vi "Reset.vi"(8 "error in (no error)":errorcluster, 11 "Debug Latest Message in":refnum<class "Debug Latest Broadcast.lvclass">) -> (0 "error out":errorcluster, 3 "Debug Latest Message out":refnum<class "Debug Latest Broadcast.lvclass">)   [LabVIEW 2020, in "Debug Latest Broadcast.lvclass"]
uses:
  Debug Latest Broadcast.lvclass
  Debug Data/Debug Data.lvclass
  Debug Latest Broadcast.lvclass/Debug Latest Broadcast.ctl
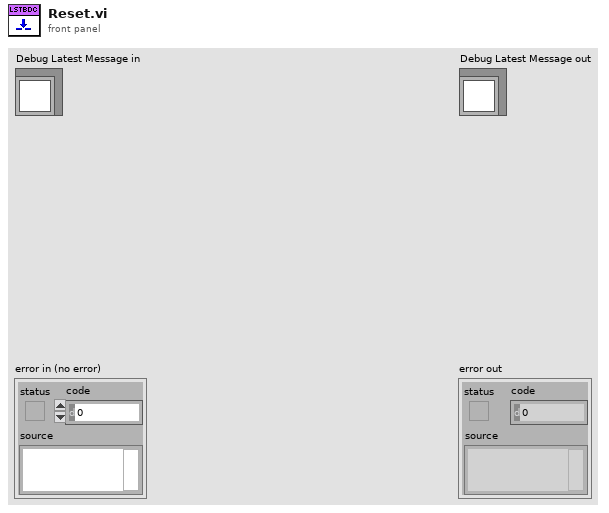
[diagram p1: front panel]
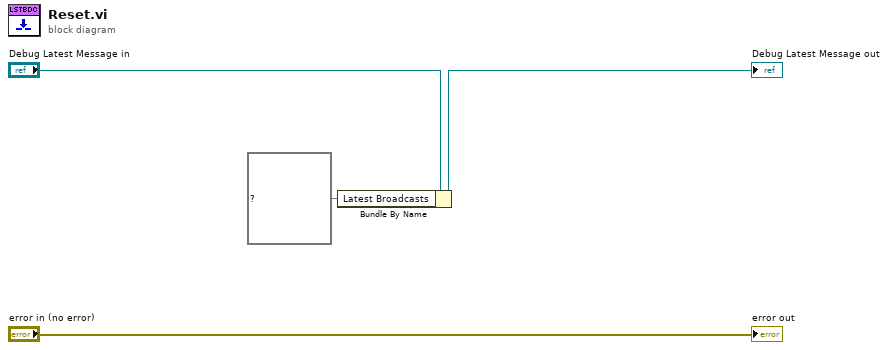
[diagram p0: block diagram]
diagram:
  n1 = Bundle By Name(cluster="Debug Latest Message in", "Latest Broadcasts"=map{string, refnum<class "Debug Data.lvclass">} {} ("Latest Messages")) -> (→"Debug Latest Message out":refnum<class "Debug Latest Broadcast.lvclass">)
  "error out" <- "error in (no error)"
